vi "AlliGator Get ROI Decay UI.vi"(7 "VI in":refnum<vi>, 8 "error in (no error)":errorcluster, 9 "ROI Descriptor":T1 {"Contours"."Type" items=["No Selection", "Point", "Line", "Rectangle", "Oval", "Polygon", "Freehand Region", "Annulus", "Unused2", "Unused3", "Broken Line", "Freehand Line", "Rotated Rectangle"]}, 10 "AlliGator Ctrl Refnums":T2, 11 "AlliGator IV DVR":refnum<data-value>) -> (0 "error out":errorcluster, 1 "Message":string, 3 "AlliGator IV DVR":refnum<data-value>)   [LabVIEW 2021, in "AlliGator Decay Analysis.lvlib" / "AlliGator Decay Processing.lvlib"]
doc: "Computes the decay at the provided ROI and adds tje computed intensity (sum of all gates) and estimated background to two separate plots in the <B>Intensity Time Trace</B> Graph."
uses:
  AlliGator Decay Processing.lvlib
  AlliGator Ctrl Refnums.ctl
  AlliGator Other Ctrl Refnums.ctl
  AlliGator State Indicator.ctl
  AlliGator Phasor Plot Ctrl Refnums.ctl
  AlliGator Phasor Graph Ctrl Refnums.ctl
  Phasor/Phasor Calibration Type.ctl
  AlliGator Dataset Ctrl Refnums.ctl
  AlliGator Displayed Image.ctl
  AlliGator Registered Events Ctrl Refnums.ctl
  AlliGator Image Histogram Control Refnums.ctl
  Histograms/Linear Histogram Options.ctl
  Histograms/Histogram Bin Option.ctl
  Histograms/Histogram Bin Position.ctl
  AlliGator Decay Fit Map Control Refnums.ctl
  Fits/IRF(X)PSED/Decay Fit Parameters & Derived Quantities List.ctl
  AlliGator Internal Variables v2.ctl
  <vilib>/vision/Image Controls.llb/IMAQ Image.ctl
  AlliGator Gate Image Set.ctl
  AlliGator FLI Dataset Type.ctl
  AlliGator Data Series Type.ctl
  AlliGator Dataset Channel.ctl
  AlliGator Gate Arithmetic.ctl
  Image/Named ROI Description.ctl
  AlliGator Decay Metadata v3.ctl
  AlliGator Decay Background Subtraction Info.ctl
  AlliGator Baseline Subtraction Method.ctl
  Graphs/XY Graph/XY Graph Plot Shift Parameters.ctl
  Graphs/XY Graph/XY Graph Plot Shift Method.ctl
  AlliGator Decay Extrapolation Parameters.ctl
  Phasor/Calibration Phasor (m, phi).ctl
  Phasor/Phasor Reference Series.ctl
  Phasor/Phasor Calibration Map v2.ctl
  Phasor/Phasor (g, s).ctl
  AlliGator Raw Phasor Plot Data v4.ctl
  Phasor/Phasor Standard Deviation Options.ctl
  AlliGator Phasor Multi-Harmonic Data.ctl
  Phasor/Phasor Harmonic Data.ctl
  AlliGator Decay Fit Options & Parameters v2.ctl
  Fits/IRF(X)PSED/Decay Fit Options v2.ctl
  Fits/Decay Convolution/Decay Model.ctl
  Fits/Residual Type.ctl
  Fits/IRF(X)PSED/Fit Weights Type.ctl
  Fits/Non-linear Fitting Method v2.ctl
  Fits/Fit Calculation Method.ctl
  Fits/Non-linear Fitting Algorithm.ctl
  AlliGator Decay Fit Parameter Constraints 2.ctl
  Fits/IRF(X)PSED/Decay Fit Parameters In List.ctl
  Fits/IRF(X)PSED/MLE Baseline Offset Type.ctl
  AlliGator Decay Preprocessing Parameters.ctl
  AlliGator Source Image.lvlib
  Graphs/XY Graph/XY Graph Add-Ons.lvlib
  AlliGator Decay Preprocessing.lvlib
  Image/Image.lvlib
  AlliGator GUI.lvlib
  Phasor/Phasor.lvlib
  AlliGator Decay Fit Parameter Map.lvlib
  AlliGator Phasor Graph.lvlib
  AlliGator Files.lvlib
  AlliGator Phasor Plot.lvlib
  Fits/Fits.lvlib
  AlliGator Decay Fit.lvlib
  AlliGator Internal Variables.lvlib
  AlliGator Settings.lvlib
  AlliGator Dual-Channel Datasets.lvlib
  Histograms/Histogram Window.lvlib
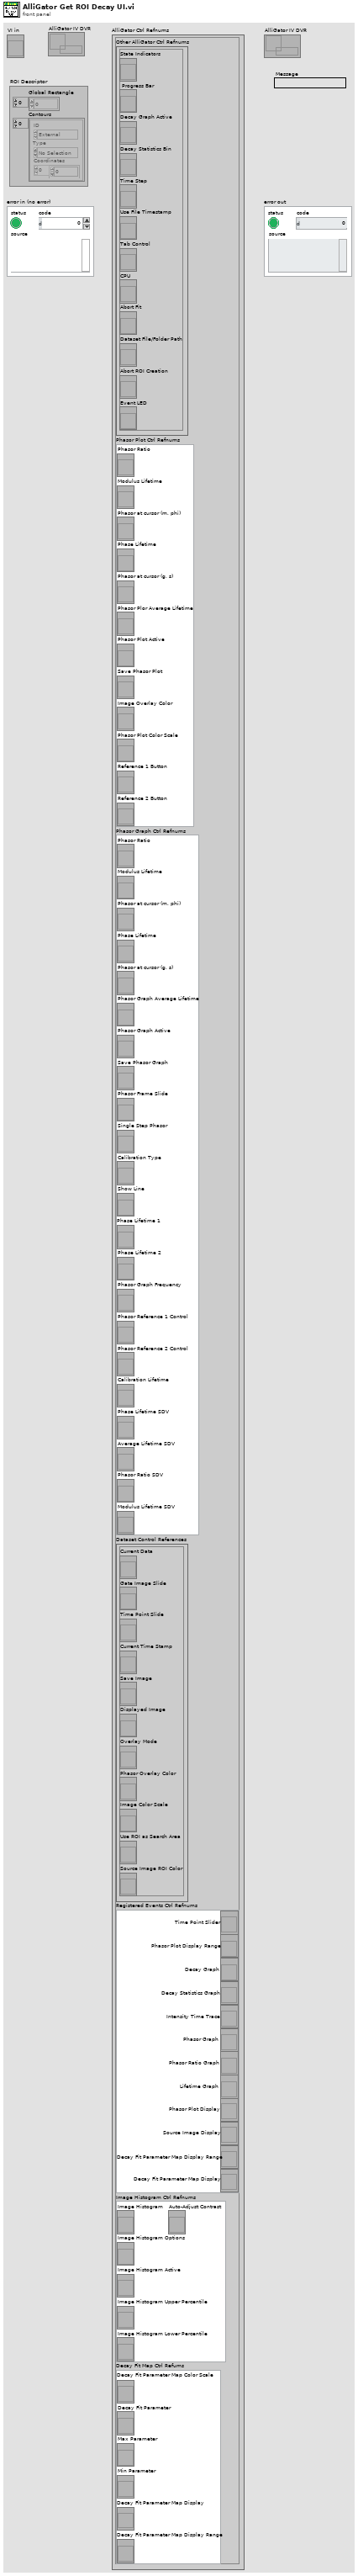
[diagram p1: front panel]
types:
  T1 = typedef "ROI Descriptor" = cluster{"Global Rectangle":i32[], "Contours":cluster{"ID":enum32{"External", "Internal"}, "Type":u32, "Coordinates":i32[]}[]}
  T2 = typedef "AlliGator GUI.lvlib/AlliGator Ctrl Refnums.ctl" = cluster{"Other AlliGator Ctrl Refnums":T3, "Phasor Plot Ctrl Refnums":T4, "Phasor Graph Ctrl Refnums":T5, "Dataset Control References":T6, "Registered Events Ctrl Refnums":T7, "Image Histogram Ctrl Refnums":T8, "Decay Fit Map Ctrl Refums":T9}
  T3 = typedef "AlliGator GUI.lvlib/AlliGator Other Ctrl Refnums.ctl" = cluster{"State Indicators":refnum<vi>, " Progress Bar":refnum<vi>, "Decay Graph Active":refnum<vi>, "Decay Statistics Bin":refnum<vi>, "Time Step":refnum<vi>, "Use File Timestamp":refnum<vi>, "Tab Control":refnum<vi>, "CPU":refnum<vi>, "Abort Fit":refnum<vi>, "Dataset File/Folder Path":refnum<vi>, "Abort ROI Creation":refnum<vi>, "Event LED":refnum<vi>}
  T4 = typedef "AlliGator GUI.lvlib/AlliGator Phasor Plot Ctrl Refnums.ctl" = cluster{"Phasor Ratio":refnum<vi>, "Modulus Lifetime":refnum<vi>, "Phasor at cursor (m, phi)":refnum<vi>, "Phase Lifetime":refnum<vi>, "Phasor at cursor (g, s)":refnum<vi>, "Phasor Plor Average Lifetime":refnum<vi>, "Phasor Plot Active":refnum<vi>, "Save Phasor Plot":refnum<vi>, "Image Overlay Color":refnum<vi>, "Phasor Plot Color Scale":refnum<vi>, "Reference 1 Button":refnum<vi>, "Reference 2 Button":refnum<vi>}
  T5 = typedef "AlliGator GUI.lvlib/AlliGator Phasor Graph Ctrl Refnums.ctl" = cluster{"Phasor Ratio":refnum<vi>, "Modulus Lifetime":refnum<vi>, "Phasor at cursor (m, phi)":refnum<vi>, "Phase Lifetime":refnum<vi>, "Phasor at cursor (g, s)":refnum<vi>, "Phasor Graph Average Lifetime":refnum<vi>, "Phasor Graph Active":refnum<vi>, "Save Phasor Graph":refnum<vi>, "Phasor Frame Slide":refnum<vi>, "Single Step Phasor":refnum<vi>, "Calibration Type":refnum<vi>, "Show Line":refnum<vi>, "Phase Lifetime 1":refnum<vi>, "Phase Lifetime 2":refnum<vi>, "Phasor Graph Frequency":refnum<vi>, "Phasor Reference 1 Control":refnum<vi>, "Phasor Reference 2 Control":refnum<vi>, "Calibration Lifetime":refnum<vi>, "Phase Lifetime SDV":refnum<vi>, "Average Lifetime SDV":refnum<vi>, "Phasor Ratio SDV":refnum<vi>, "Modulus Lifetime SDV":refnum<vi>}
  T6 = typedef "AlliGator GUI.lvlib/AlliGator Dataset Ctrl Refnums.ctl" = cluster{"Current Data":refnum<vi>, "Gate Image Slide":refnum<vi>, "Time Point Slide":refnum<vi>, "Current Time Stamp":refnum<vi>, "Save Image":refnum<vi>, "Displayed Image":refnum<vi>, "Overlay Mode":refnum<vi>, "Phasor Overlay Color":refnum<vi>, "Image Color Scale":refnum<vi>, "Use ROI as Search Area":refnum<vi>, "Source Image ROI Color":refnum<vi>}
  T7 = typedef "AlliGator GUI.lvlib/AlliGator Registered Events Ctrl Refnums.ctl" = cluster{"Time Point Slider":refnum<vi>, "Phasor Plot Display Range":refnum<vi>, "Decay Graph":refnum<vi>, "Decay Statistics Graph":refnum<vi>, "Intensity Time Trace":refnum<vi>, "Phasor Graph":refnum<vi>, "Phasor Ratio Graph":refnum<vi>, "Lifetime Graph":refnum<vi>, "Phasor Plot Display":refnum<vi>, "Source Image Display":refnum<vi>, "Decay Fit Parameter Map Display Range":refnum<vi>, "Decay Fit Parameter Map Display":refnum<vi>}
  T8 = typedef "AlliGator GUI.lvlib/AlliGator Image Histogram Control Refnums.ctl" = cluster{"Image Histogram":refnum<vi>, "Image Histogram Options":refnum<vi>, "Image Histogram Active":refnum<vi>, "Image Histogram Upper Percentile":refnum<vi>, "Image Histogram Lower Percentile":refnum<vi>, "Auto-Adjust Contrast":refnum<vi>}
  T9 = typedef "AlliGator Decay Fit Parameter Map.lvlib/AlliGator Decay Fit Map Control Refnums.ctl" = cluster{"Decay Fit Parameter Map Color Scale":refnum<vi>, "Decay Fit Parameter":refnum<vi>, "Max Parameter":refnum<vi>, "Min Parameter":refnum<vi>, "Decay Fit Parameter Map Display":refnum<vi>, "Decay Fit Parameter Map Display Range":refnum<vi>}
  T10 = typedef "Image.lvlib/Image Control Refnum.ctl" = refnum<vi>
  T11 = typedef "AlliGator Decay Analysis.lvlib/AlliGator ROI Decay Addl Data.ctl" = cluster{"ROI Center":cluster{"X":i32, "Y":i32}, "Current Dataset":i32, "Time Stamp (s)":dbl, "Bkgd-subtracted Intensity":dbl, "Background (ROI)":dbl}
  T12 = typedef "AlliGator Phasor Graph.lvlib/AlliGator Decay Metadata v3.ctl" = cluster{"ROI Descriptor":T1, "ROI Center":cluster{"X":i32, "Y":i32}, "Decay Background Subtraction Info":T13, "Decay Reverted":bool, "Decay Smoothened":bool, "Decay Straightened":bool, "Fitted Tau (Decay Straightening)":dbl, "Decay Shift Parameters":T15, "Decay Shifted":bool, "Decay Extrapolated":bool, "Decay Extrapolation Parameters":T17, "Decay Normalized":bool, "Fold Decay":bool, "# Folds":u32}
  T13 = typedef "AlliGator Decay Analysis.lvlib/AlliGator Decay Preprocessing.lvlib/AlliGator Decay Background Subtraction Info.ctl" = cluster{"Laser Period":dbl[unit], "Gate Duration":dbl[unit], "Baseline Subtraction Method":T14, "Background Definition Range":cluster{"Min Gate":dbl[unit], "Max Gate":dbl[unit]}, "Total Intensity w/o Bkgd Subtraction":dbl, "Bkgd-subtracted Intensity (exp)":dbl, "# Data Points":i32, "Background/Gate":dbl, "Fitted Lifetime":dbl[unit], "Bkgd-subtracted Intensity (theo)":dbl}
  T14 = typedef "AlliGator Decay Analysis.lvlib/AlliGator Decay Preprocessing.lvlib/AlliGator Baseline Subtraction Method.ctl" = enum16{"Mean", "Min", "Square Gated Single-Exponential", "File", "Constant"}
  T15 = typedef "XY Graph Add-Ons.lvlib/XY Graph Plot Shift Parameters.ctl" = cluster{"Type":T16, "Shift":dbl[unit], "Threshold":dbl, "Rotate":bool}
  T16 = typedef "XY Graph Add-Ons.lvlib/XY Graph Plot Shift Method.ctl" = enum16{"Default", "CFD", "Threshold", "Cross-Correlation"}
  T17 = typedef "AlliGator Decay Analysis.lvlib/AlliGator Decay Preprocessing.lvlib/AlliGator Decay Extrapolation Parameters.ctl" = cluster{"Additional Points":u32, "Head Fraction":dbl, "Fitted Tau":dbl, "Use Periodicity":bool, "Use Cursors":bool, "Tail Fraction":dbl}
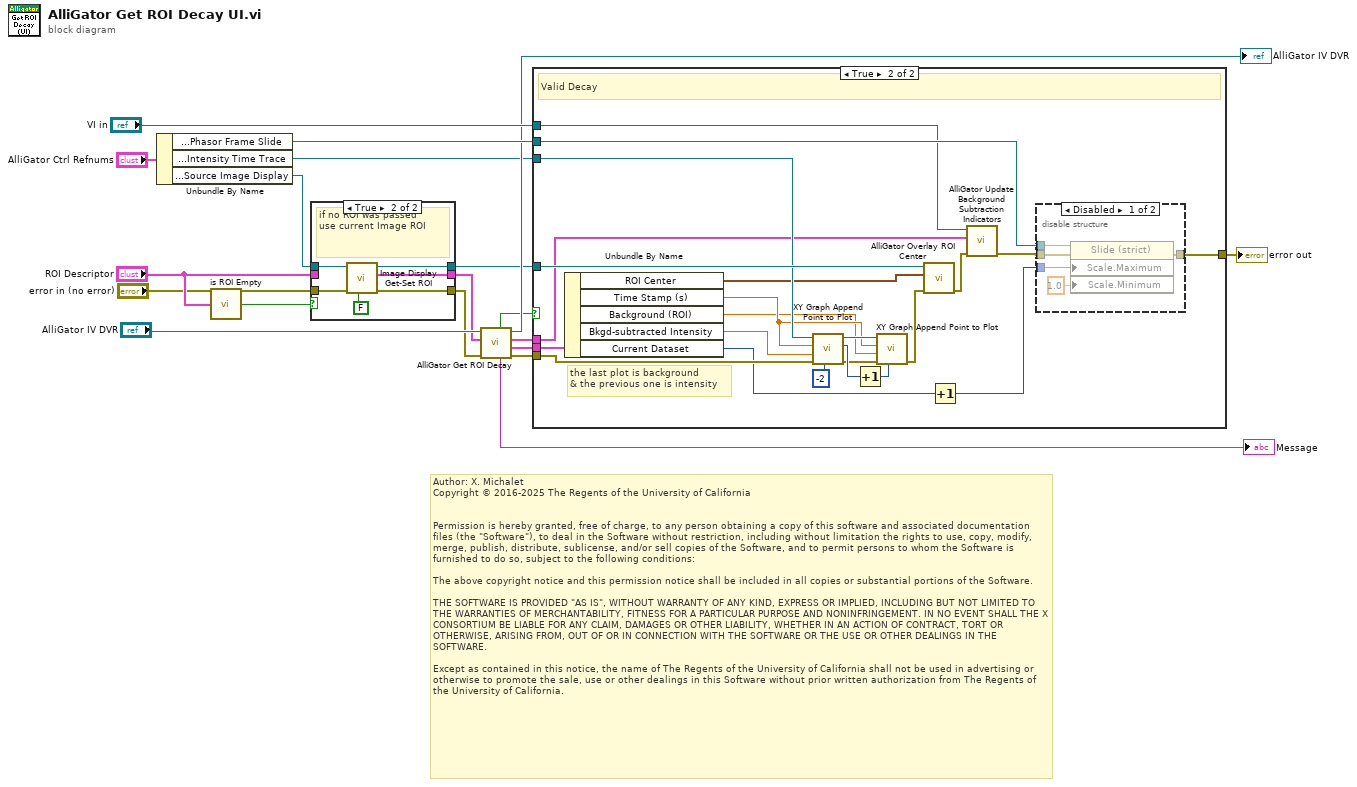
[diagram p0: block diagram]
diagram:
  # "Author: X. Michalet\nCopyright © 2016-2025 The Regents of the University of California\n \n\nPermission is hereby granted, free of charge, to any person obtaining a copy of this software and associated documentation files (the \"Software\"), to deal in the Software without restriction, including without limitation the rights to use, copy, modify, merge, publish, distribute, sublicense, and/or sell copies of the Software, and to permit persons to whom the Software is furnished to do so, subject to the following conditions:\n\nThe above copyright notice and this permission notice shall be included in all copies or substantial portions of the Software.\n\nTHE SOFTWARE IS PROVIDED \"AS IS\", WITHOUT WARRANTY OF ANY KIND, EXPRESS OR IMPLIED, INCLUDING BUT NOT LIMITED TO THE WARRANTIES OF MERCHANTABILITY, FITNESS FOR A PARTICULAR PURPOSE AND NONINFRINGEMENT. IN NO EVENT SHALL THE X CONSORTIUM BE LIABLE FOR ANY CLAIM, DAMAGES OR OTHER LIABILITY, WHETHER IN AN ACTION OF CONTRACT, TORT OR OTHERWISE, ARISING FROM, OUT OF OR IN CONNECTION WITH THE SOFTWARE OR THE USE OR OTHER DEALINGS IN THE SOFTWARE.\n\nExcept as contained in this notice, the name of The Regents of the University of California shall not be used in advertising or otherwise to promote the sale, use or other dealings in this Software without prior written authorization from The Regents of the University of California."
  n1 = Unbundle By Name("AlliGator Ctrl Refnums") -> ("Phasor Graph Ctrl Refnums.Phasor Frame Slide"=w18:refnum<vi>, "Registered Events Ctrl Refnums.Intensity Time Trace"=w9:refnum<vi>, "Registered Events Ctrl Refnums.Source Image Display"=w11:refnum<vi>)
  n2 = call "is ROI Empty.vi"("Current ROI Descriptor"="ROI Descriptor") -> ("Empty ROI?"=w2:bool)  [unwired: 8 in]
  n3 = case shown="True" w2 {
    tunnel: w11 -> [w22 w27]
    tunnel: [w22 w26] -> w12
    tunnel: [w21 w25] -> w10
    tunnel: [w20 w24] -> w8
    tunnel: "ROI Descriptor" -> [w21 _]
    tunnel: "error in (no error)" -> [w20 w23]
    frame False {
      # "not an empty ROI"
    }
    frame True {
      # "if no ROI was passed\nuse current Image ROI"
      n4 = call "Image Display Get-Set ROI.vi"("Get(F)/Set"=FALSE ("Get(F)/Set(T)"), "Error In"=w23, "Image Display Refnum"=w27) -> ("Error Out"=w24:errorcluster, "ROI Descriptor out"=w25:T1, "Image Display Refnum (dup)"=w26:T10)  [unwired: 4 in, 2 out]
    }
  }
  n5 = call "AlliGator Get ROI Decay.vi"("error in (no error)"=w8, "ROI Descriptor"=w10, "AlliGator Internal Variables DVR"="AlliGator IV DVR") -> ("Error Out"=w19:errorcluster, "ROI Decay Add'l Data"=w6:T11, "Decay Metadata"=w7:T12, "AlliGator Internal Variables DVR"=→"AlliGator IV DVR":refnum<data-value>, "Message"=→"Message":string, "Valid Decay?"=w4:bool)  [unwired: 3 in]
  n6 = case shown="True" w4 {
    tunnel: w19 -> [w29 w50]
    tunnel: w18 -> [_ w47]
    tunnel: "VI in" -> [_ w46]
    tunnel: [w29 w39] -> w13
    tunnel: w12 -> [_ w38]
    tunnel: w9 -> [_ w37]
    tunnel: w7 -> [_ w32]
    tunnel: w6 -> [_ w31]
    frame False {
      # "Invalid Decay"
    }
    frame True {
      # "the last plot is background\n& the previous one is intensity"
      # "Valid Decay"
      n7 = Unbundle By Name(w31) -> ("ROI Center"=w36:cluster{"X":i32, "Y":i32}, "Time Stamp (s)"=w35:dbl, "Background (ROI)"=w34:dbl, "Bkgd-subtracted Intensity"=w33:dbl, "Current Dataset"=w30:i32)
      n8 = call "XY Graph Append Point to Plot.vi"("Plot ID (-1: last)"=-2, "error in (no error)"=w50, "y"=w33, "x"=w35, "XYGraph in"=w37) -> ("error out"=w41:errorcluster, "Actual Plot ID"=w42:i32)  [unwired: 3 in, 2 out]
      n9 = Increment(x=w42) -> (x+1=w43:i32)
      n10 = call "XY Graph Append Point to Plot.vi"("Plot ID (-1: last)"=w43, "error in (no error)"=w41, "y"=w34, "x"=w35, "XYGraph in"=w37) -> ("error out"=w40:errorcluster)  [unwired: 3 in, 3 out]
      n11 = call "AlliGator Overlay ROI Center.vi"("error in (no error)"=w40, "ROI Center"=w36, "Display Image Control Refnum"=w38) -> ("Error Out"=w45:errorcluster)  [unwired: 8 in]
      n12 = Increment(x=w30) -> (x+1=w49:i32)
      n13 = call "AlliGator Update Background Subtraction Indicators.vi"("Error In"=w45, "Decay Metadata"=w32, "AlliGator Ref"=w46) -> ("Error Out"=w48:errorcluster)  [unwired: 8 in]
      n14 = disable-structure shown="Disabled" {
        disable-tunnel: w49 -> [w54 _]
        disable-tunnel: w48 -> [w53 w56]
        disable-tunnel: w47 -> [w52 _]
        disable-tunnel: [w51 w56] -> w39
        frame Disabled {
          n15 = property class="Slide (strict)"(reference=w52, error in=w53, "Scale.Maximum"=w54, "Scale.Minimum"=1.0 ("Scale.Range:Minimum")) -> (error out=w51:errorcluster)  [unwired: 1 out]
        }
        frame Enabled {
        }
      }
    }
  }
  "error out" <- w13
